vi "Send Configure Start Trigger [STT].vi"(6 "Trigger Slope (Positive)":i32(ring) caption="trigger slope (Positive)" items=["Positive", "Negative", "Either"], 7 "Message Priority (Normal)":T1=enum."Normal", 8 "error in (no error)":errorcluster, 9 "Trigger Source (None)":string(combo) caption="trigger source (None)", 10 "Channel Name (\"\")":string="CHANNEL1" caption="channel name (\"CHANNEL1\")", 11 "Message Enqueuer":refnum<class "Message Enqueuer.lvclass">) -> (0 "error out":errorcluster, 3 "Message Enqueuer out":refnum<class "Message Enqueuer.lvclass">)   [LabVIEW 2016, in "CS++Fgen.lvlib" / "Configure Start Trigger [STT] Msg.lvclass"]
doc: "Sends the <B>CS++Fgen.lvlib:Configure Start Trigger [STT] Msg.lvclass</B> message.\n\n<B>CS++Fgen.lvlib:CS++Fgen.lvclass:Configure Start Trigger [STT].vi</B> Description:\n\nThis VI configures the properties that control the function generator's start trigger. These properties are the start trigger source and slope.\n\nA start trigger initiates generation of a waveform or sequence. \n\nNote:\n\n(1) This VI is part of the IviFgenStartTrigger [STT] extension group."
uses:
  Configure Start Trigger [STT] Msg.lvclass
  <vilib>/ActorFramework/Message Enqueuer/Message Enqueuer.lvclass
  <vilib>/ActorFramework/Message Enqueuer/Message Priority.ctl
  C:/Program Files (x86)/National Instruments/LabVIEW 2016/vi.lib/ActorFramework/Message/Message.lvclass
  Configure Start Trigger [STT] Msg.lvclass/Configure Start Trigger [STT] Msg.ctl
  <vilib>/ActorFramework/Message Enqueuer/Message Enqueuer.lvclass/Message Enqueuer.ctl
  <vilib>/ActorFramework/Message Priority Queue/Priority Enqueue.vi
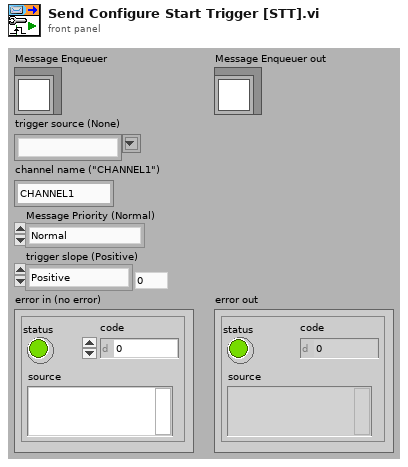
[diagram p1: front panel]
types:
  T1 = typedef "Actor Framework.lvlib/Message Enqueuer.lvclass/Message Priority.ctl" = enum16{"Low", "Normal", "High"}
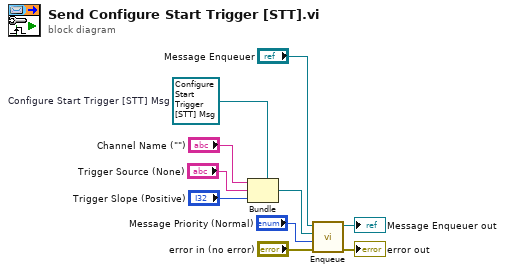
[diagram p0: block diagram]
diagram:
  w4 = refnum<class "Configure Start Trigger [STT] Msg.lvclass"> refnum  # Configure Start Trigger [STT] Msg
  n1 = Bundle(cluster=w4, "Channel Name (\"\")", "Trigger Source (None)", "Trigger Slope (Positive)") -> (w7:refnum<class "Configure Start Trigger [STT] Msg.lvclass">)
  n2 = call <vilib>:"Enqueue.vi"("error in (no error)"="error in (no error)", "Message Priority (Normal)"="Message Priority (Normal)", "Message"=w7, "Message Enqueuer in"="Message Enqueuer") -> ("error out"=→"error out":errorcluster, "Message Enqueuer out"=→"Message Enqueuer out":refnum<class "Message Enqueuer.lvclass">)  [unwired: 6 in]
